vi "Create Evaluations.vi"(8 "error in (no error)":errorcluster, 11 "Skyworks - 2G PVT in":refnum<class "Skyworks - PVT.lvclass">) -> (0 "error out":errorcluster, 1 "Evaluations Out":T1[](array[typedef]) {"Low Limit" format="%#_13g"; "SI Scaling" items=["femto"=-15, "pico"=-12, "nano"=-9, "micro"=-6, "milli"=-3, "percent"=-2, ""=0, "kilo"=3, "mega"=6, "giga"=9, "tera"=12]}, 3 "Skyworks - 2G PVT out":refnum<class "Skyworks - PVT.lvclass">)   [LabVIEW 2018, in "Skyworks PVT.lvlib" / "Skyworks - PVT.lvclass"]
uses:
  Skyworks - PVT.lvclass
  C:/Sequence Automation/Plugins/Measurement Interface.lvlibp/Measurement Interface.lvclass
  Plugins/TestStand API Tools (TSAT).lvlibp/Evaluation Actions/Includes/Controls/TSAT Evaluation.ctl
  Plugins/TestStand API Tools (TSAT).lvlibp/Evaluation Actions/Includes/Controls/TSAT Eval SI Unit Scaling.ctl
  Plugins/TestStand API Tools (TSAT).lvlibp/Evaluation Actions/Includes/Controls/TSAT Evaluation Type.ctl
  Skyworks - PVT.lvclass/Skyworks - PVT.ctl
  Plugins/Measurement Interface.lvlibp/Private Methods/Measurement Name/Read Measurement Name.vi
  Plugins/SeqAuto Evaluations.lvlibp/Skyworks/2G_PVT/Skyworks_2G_PVT.lvclass
  Plugins/TestStand API Tools (TSAT).lvlibp/Evaluation Actions/TSAT Evaluation Actions.lvlib
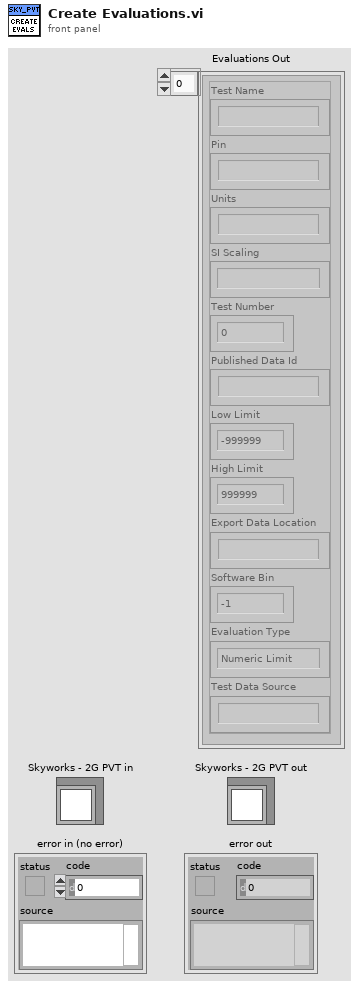
[diagram p1: front panel]
types:
  T1 = typedef "TestStand API Tools (TSAT).lvlibp/TSAT Evaluation Actions.lvlib/TSAT Evaluation.ctl" = cluster{"Test Name":string, "Pin":string, "Units":string, "SI Scaling":T2, "Test Number":i32, "Published Data Id":string, "Low Limit":dbl, "High Limit":dbl, "Export Data Location":string, "Software Bin":i64, "Evaluation Type":T3, "Test Data Source":string}
  T2 = typedef "TestStand API Tools (TSAT).lvlibp/TSAT Evaluation Actions.lvlib/TSAT Eval SI Unit Scaling.ctl" = i16
  T3 = typedef "TestStand API Tools (TSAT).lvlibp/TSAT Evaluation Actions.lvlib/TSAT Evaluation Type.ctl" = enum16{"Numeric Limit", "Pass/Fail", "None"}
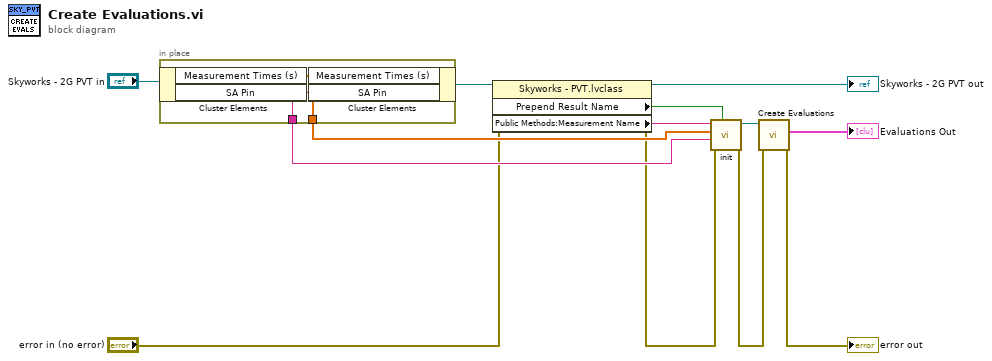
[diagram p0: block diagram]
diagram:
  n1 = in-place {
    in-place-border: [w15] -> w9
    in-place-border: [w14] -> w8
    n2 = in-place-cluster #1("Skyworks - 2G PVT in") -> ("Measurement Times (s)"=w15:dbl[], "SA Pin"=w14:string)
    n3 = in-place-cluster #1("Measurement Times (s)"=w15, "SA Pin"=w14) -> (w10:refnum<class "Skyworks - PVT.lvclass">)
  }
  n4 = property class="Skyworks - PVT.lvclass"(reference=w10, error in="error in (no error)") -> (reference out=→"Skyworks - 2G PVT out":refnum<class "Skyworks - PVT.lvclass">, error out=w4:errorcluster, "Prepend Result Name"=w12:bool, "Public Methods:Measurement Name"=w11:string)
  n5 = call "init.vi"("Prepend Result Name"=w12, "error in (no error)"=w4, "SA Pin"=w8, "Measurement Times (s)"=w9, "Measurement Name"=w11) -> ("error out"=w3:errorcluster, "Skyworks_2G_PVT out"=w13:refnum<class "Skyworks_2G_PVT.lvclass">)  [unwired: 5 in]
  n6 = call-dynamic "Create Evaluations.vi"("error in (no error)"=w3, "IEvaluation in"=w13) -> ("error out"=→"error out":errorcluster, "Evaluations Out"=→"Evaluations Out":T1[])  [unwired: 7 in, 1 out]
